vi "CetoniConditionalRefill.vi"(0 "object in":refnum<class "Application.lvclass">, 1 "refill below level":dbl=1000.0, 2 "Refill Rate(ul/min)":dbl=10000.0, 3 "Empty Rate":dbl, 5 "error in (no error)":errorcluster, 7 "Wait After cond Refill":dbl, 8 "Timeout Refill":dbl=20.0 caption="TimeOut Refill", 9 "Empty Before Refilling":bool, 11 "Turn OFF WFG During Refill":bool) -> (14 "object out":refnum<class "Application.lvclass">, 19 "error out":errorcluster)   [LabVIEW 2023, in "Application.lvclass"]
uses:
  Application.lvclass
  CetoniPump_class/CetoniPump.lvclass
  AFG3022B_OJ_class/AFG3022B_OJ.lvclass
  Application.lvclass/Application.ctl
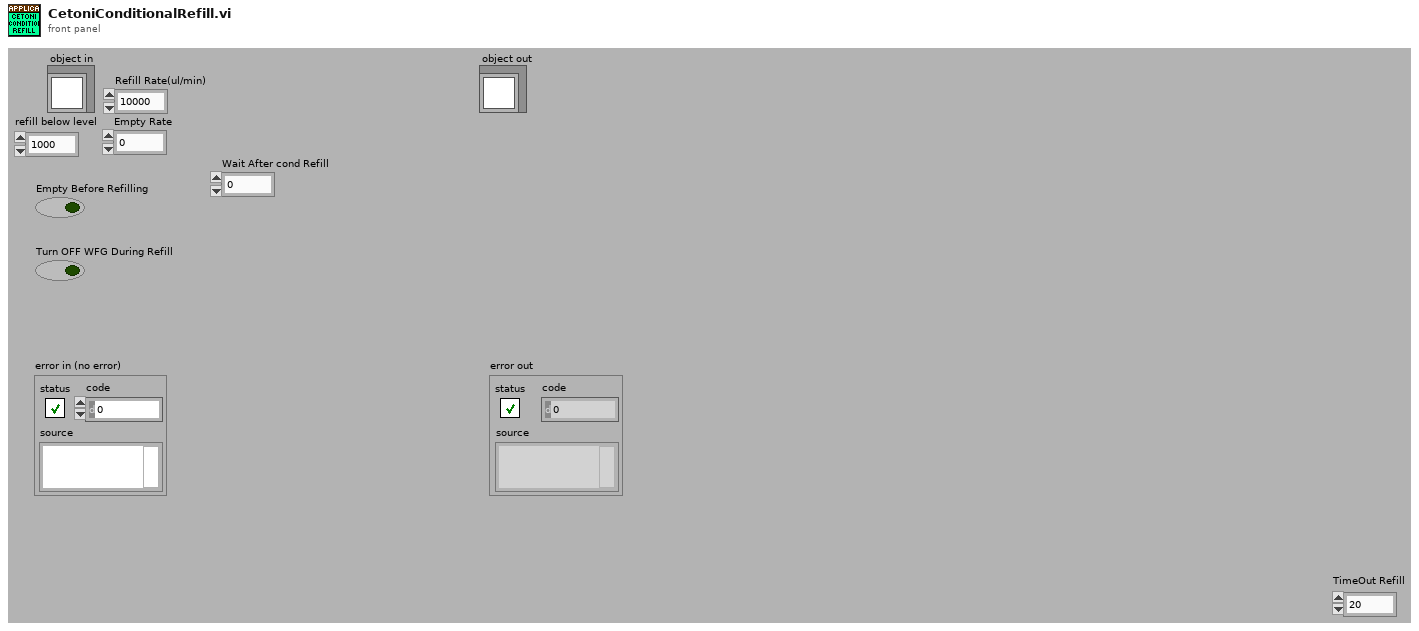
[diagram p1: front panel]
types:
  T1 = cluster{"index":i32, "Level(ml)":dbl, "Flow":dbl}
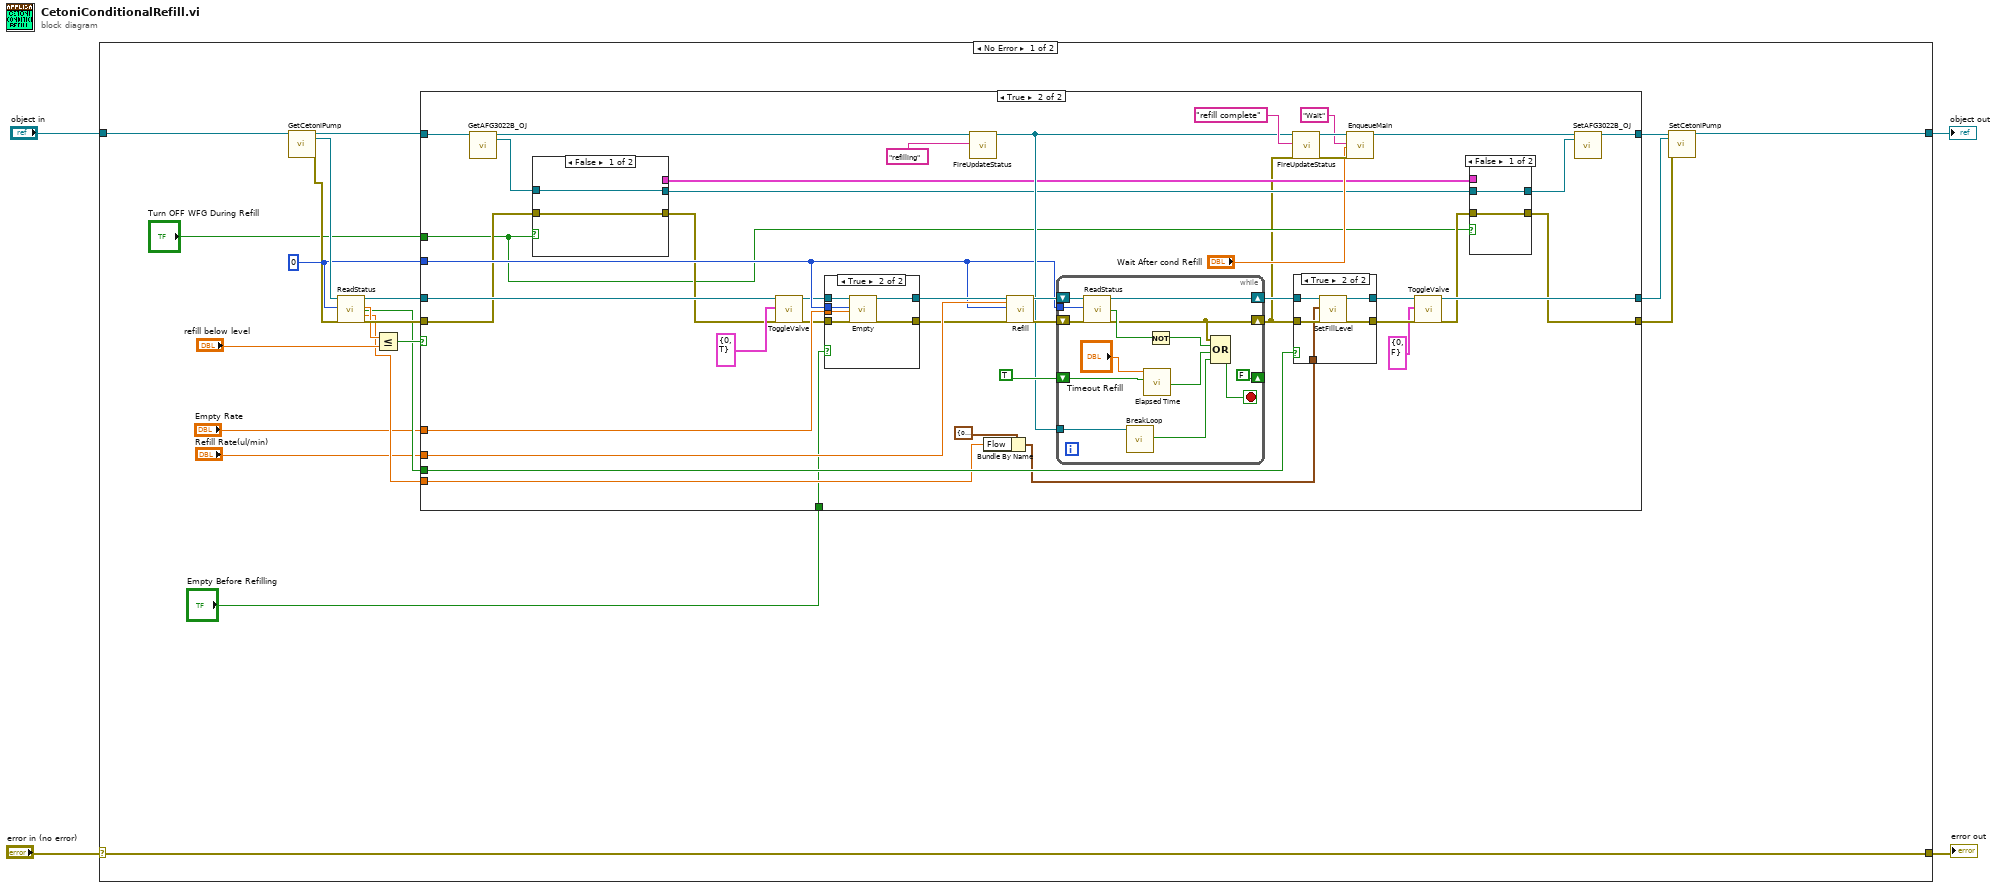
[diagram p0: block diagram]
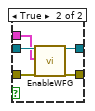
[diagram p3: hidden frame]
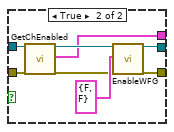
[diagram p4: hidden frame]
diagram:
  n1 = case shown="No Error" "error in (no error)" {
    selector: "error in (no error)" -> [w25 w119]
    tunnel: [w25 w119] -> w3
    tunnel: [w9 w118] -> w1
    tunnel: "object in" -> [w8 w118]
    frame No Error {
      w23 = 0 ("index")
      n2 = call-dynamic "GetCetoniPump.vi"("object in"=w8) -> ("object out"=w14:refnum<class "Application.lvclass">, "CetoniPump"=w24:refnum<class "CetoniPump.lvclass">, "error out"=w16:errorcluster)  [unwired: 16 in]
      n3 = call-dynamic "ReadStatus.vi"("object in"=w24, "index"=w23, "error in (no error)"=w16) -> ("object out"=w22:refnum<class "CetoniPump.lvclass">, "Fill Level"=w19:dbl, "Is pumping"=w12:bool, "Actual Flow Rate"=w11:dbl, "error out"=w21:errorcluster)  [unwired: 12 in]
      n4 = Less Or Equal?(x=w19, y="refill below level") -> (x <= y?=w20:bool)
      n5 = case shown="True" w20 {
        tunnel: w23 -> [_ w51]
        tunnel: w22 -> [w28 w47]
        tunnel: w21 -> [w27 w38]
        tunnel: [w28 w44] -> w17
        tunnel: [w27 w32] -> w15
        tunnel: w14 -> [w26 w55]
        tunnel: [w26 w35] -> w13
        tunnel: w12 -> [_ w61]
        tunnel: w11 -> [_ w59]
        tunnel: "Refill Rate(ul/min)" -> [_ w57]
        tunnel: "Empty Rate" -> [_ w52]
        tunnel: "Empty Before Refilling" -> [_ w50]
        tunnel: "Turn OFF WFG During Refill" -> [_ w31]
        frame False {
        }
        frame True {
          n6 = call-dynamic "GetAFG3022B_OJ.vi"("object in"=w55) -> ("object out"=w41:refnum<class "Application.lvclass">, "AFG3022B_OJ"=w39:refnum<class "AFG3022B_OJ.lvclass">)  [unwired: 16 in, 1 out]
          n7 = case shown="False" w31 {
            tunnel: [w79 w87] -> w40
            tunnel: w39 -> [w80 w86]
            tunnel: w38 -> [w79 w84]
            tunnel: [w80 w82] -> w37
            tunnel: [_ w81] -> w30
            frame False {
            }
            frame True {
              n8 = call-dynamic "GetChEnabled.vi"("object in"=w86, "error in (no error)"=w84) -> ("object out"=w83:refnum<class "AFG3022B_OJ.lvclass">, "Ch Enabled"=w81:cluster{"Ch1Enabled":bool, "Ch2Enabled":bool}, "error out"=w85:errorcluster)  [unwired: 15 in]
              n9 = call-dynamic "EnableWFG.vi"("object in"=w83, "Enable Channels"=cluster{"Ch1":bool, "Ch2":bool} {"Ch1"=FALSE, "Ch2"=FALSE}, "error in (no error)"=w85) -> ("object out"=w82:refnum<class "AFG3022B_OJ.lvclass">, "error out"=w87:errorcluster)  [unwired: 15 in]
            }
          }
          n10 = call-dynamic "ToggleValve.vi"("object in"=w47, "ValveControl"=cluster{"index":i32, "Valve Position":bool} {"index"=0, "Valve Position"=TRUE}, "error in (no error)"=w40) -> ("object out"=w48:refnum<class "CetoniPump.lvclass">, "error out"=w46:errorcluster)  [unwired: 15 in]
          n11 = case shown="True" w50 {
            tunnel: [w90 w96] -> w54
            tunnel: w48 -> [w90 w95]
            tunnel: [w89 w94] -> w53
            tunnel: w46 -> [w89 w93]
            tunnel: w52 -> [_ w92]
            tunnel: w51 -> [_ w91]
            frame False {
            }
            frame True {
              n12 = call-dynamic "Empty.vi"("object in"=w95, "index"=w91, "Empty Rate"=w92, "error in (no error)"=w93) -> ("object out"=w96:refnum<class "CetoniPump.lvclass">, "error out"=w94:errorcluster)  [unwired: 14 in]
            }
          }
          n13 = call-dynamic "FireUpdateStatus.vi"("object in"=w41, "Status"="refilling") -> ("object out"=w56:refnum<class "Application.lvclass">)  [unwired: 16 in, 1 out]
          n14 = Bundle By Name(cluster=T1 {"index"=0, "Level(ml)"=0.0, "Flow"=0.0} ("GoToLevelSettings"), "Flow"=w59) -> (w58:T1)
          n15 = call-dynamic "Refill.vi"("object in"=w54, "Refill Rate"=w57, "index"=w51, "error in (no error)"=w53) -> ("object out"=w71:refnum<class "CetoniPump.lvclass">, "error out"=w70:errorcluster)  [unwired: 14 in]
          n16 = while {
            tunnel: w51 -> [w116]
            shift-right: [w110] -> w62
            shift-left: w71 -> [w117]
            shift-right: [w105] -> w29
            shift-left: w70 -> [w115]
            shift-right: [FALSE] -> _
            shift-left: TRUE -> [w112]
            tunnel: w56 -> [w109]
            stop <- w104 stop-if-true
            n17 = call-dynamic "ReadStatus.vi"("object in"=w117, "index"=w116, "error in (no error)"=w115) -> ("object out"=w110:refnum<class "CetoniPump.lvclass">, "Is pumping"=w113:bool, "error out"=w105:errorcluster)  [unwired: 12 in, 2 out]
            n18 = call-dynamic "BreakLoop.vi"("object in"=w109) -> ("Abort"=w108:bool)  [unwired: 16 in, 2 out]
            n19 = call "Elapsed Time"("Time Target (s)"="Timeout Refill", "Reset"=w112) -> ("Time has Elapsed"=w106:bool)  [unwired: 10 in, 7 out]
            n20 = Not(x=w113) -> (.not. x?=w107:bool)
            n21 = Compound Arithmetic op=OR(w105, w107, w106, w108) -> (w104:bool)
          }
          n22 = call-dynamic "FireUpdateStatus.vi"("object in"=w56, "Status"="refill complete", "error in (no error)"=w29) -> ("object out"=w65:refnum<class "Application.lvclass">, "error out"=w66:errorcluster)  [unwired: 15 in]
          n23 = case shown="True" w61 {
            tunnel: w62 -> [w98 w103]
            tunnel: [w98 w102] -> w45
            tunnel: w29 -> [w97 w101]
            tunnel: w58 -> [_ w100]
            tunnel: [w97 w99] -> w43
            frame False {
            }
            frame True {
              n24 = call-dynamic "SetFillLevel.vi"("object in"=w103, "GoToLevelSettings"=w100, "error in (no error)"=w101) -> ("object out"=w102:refnum<class "CetoniPump.lvclass">, "error out"=w99:errorcluster)  [unwired: 12 in, 3 out]
            }
          }
          n25 = call-dynamic "EnqueueMain.vi"("object in"=w65, "Message"="Wait" ("Status"), "Message Data"="Wait After cond Refill", "error in (no error)"=w66) -> ("object out"=w36:refnum<class "Application.lvclass">)  [unwired: 14 in, 1 out]
          n26 = call-dynamic "ToggleValve.vi"("object in"=w45, "ValveControl"=cluster{"index":i32, "Valve Position":bool} {"index"=0, "Valve Position"=FALSE}, "error in (no error)"=w43) -> ("object out"=w44:refnum<class "CetoniPump.lvclass">, "error out"=w33:errorcluster)  [unwired: 15 in]
          n27 = case shown="False" w31 {
            tunnel: w37 -> [w72 w78]
            tunnel: [w72 w77] -> w34
            tunnel: w33 -> [w73 w76]
            tunnel: [w73 w75] -> w32
            tunnel: w30 -> [_ w74]
            frame False {
            }
            frame True {
              n28 = call-dynamic "EnableWFG.vi"("object in"=w78, "Enable Channels"=w74, "error in (no error)"=w76) -> ("object out"=w77:refnum<class "AFG3022B_OJ.lvclass">, "error out"=w75:errorcluster)  [unwired: 15 in]
            }
          }
          n29 = call-dynamic "SetAFG3022B_OJ.vi"("object in"=w36, "AFG3022B_OJ"=w34) -> ("object out"=w35:refnum<class "Application.lvclass">)  [unwired: 16 in, 1 out]
        }
      }
      n30 = call-dynamic "SetCetoniPump.vi"("object in"=w13, "CetoniPump"=w17, "error in (no error)"=w15) -> ("object out"=w9:refnum<class "Application.lvclass">)  [unwired: 15 in, 1 out]
    }
    frame Error {
    }
  }
  "error out" <- w3
  "object out" <- w1
